vi "get one frame - subvi.vi"(9 "Image Height":i32, 10 "Image Width":i32) -> (3 "Image Array":i32[][](array[numeric]))   [LabVIEW 2014]
uses:
  Library Files - Andor and MadCity/Andorlib/atmcd32d.lvlib
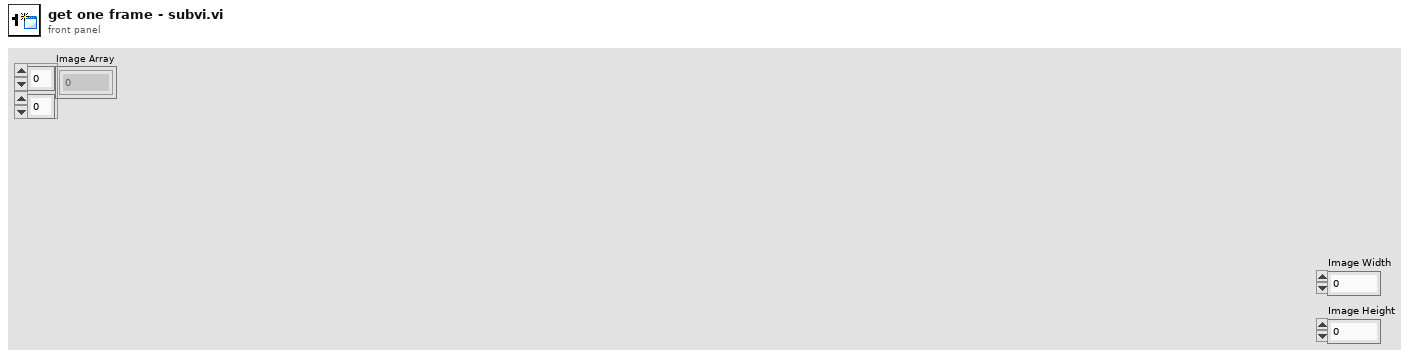
[diagram p1: front panel]
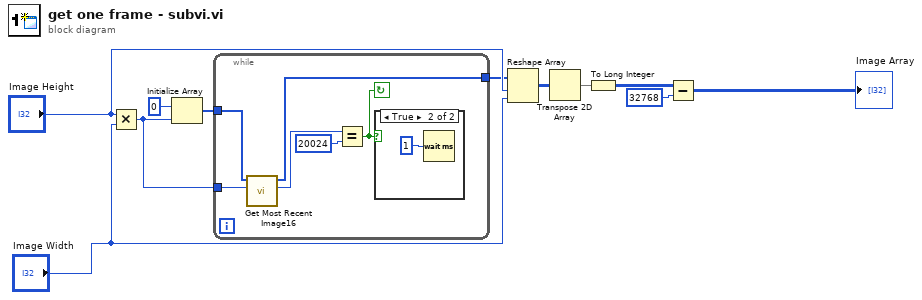
[diagram p0: block diagram]
diagram:
  n1 = Multiply(x="Image Height", y="Image Width") -> (x*y=w6:i32)
  n2 = Initialize Array(u16 0, w6) -> (w7:u16[])
  n3 = while {
    tunnel: w7 -> [w14]
    tunnel: w6 -> [w13]
    tunnel: [w12] -> w5
    stop <- w15 continue-if-true
    n4 = call "Get Most Recent Image16.vi"("size"=w13, "Array 2"=w14) -> ("function return"=w16:u32, "Array"=w12:u16[])  [unwired: 7 in, 1 out]
    n5 = Equal?(x=w16, y=20024) -> (x = y?=w15:bool)
    n6 = case shown="True" w15 {
      frame False {
      }
      frame True {
        n7 = Wait (ms)(milliseconds to wait=u32 1) -> ()  [unwired: 1 out]
      }
    }
  }
  n8 = Reshape Array(w5, "Image Height", "Image Width") -> (w2:u16[][])
  n9 = Transpose 2D Array(2D array=w2) -> (transposed array=w1:u16[][])
  n10 = To Long Integer(number=w1) -> (32bit integer=w4:i32[][])
  n11 = Subtract(x=w4, y=32768) -> (x-y=→"Image Array":i32[][])
